vi "Settings Dialog.vi"(8 "error in (no error)":errorcluster caption="错误输入（无错误）", 11 "Settings in":T10={"Hardware Configuration"={"电压读取设置"={"DAQmx Channel"="", "Max Input"=0.0, "Min Input"=0.0, "Sample Rate"=0.0, "Sample Number"=0, "DAQmx Task"="", "device in"=""}, "角度传感器设置"={"counter"="Dev1/ctr0", "units"=10146, "分辨率"=0, "初始角度"=0.0, "DecodingType"=10092, "A相端口"="/Dev1/PFI8", "B相端口"="/Dev1/PFI8", "task in"=""}}, "Logging Configuration"={"Log File Base Path"=path "", "电压传感器转换率"=[], "电压传感器本底"=[]}, "Action Configuration"={"PLC设置"={"ActLogicalStationNumber"=9600, "ActUtlType"=refnum}, "动作设置"={"自动跳法测试动作"={"夹紧/松阀总"={"变量类型"=2, "PLC地址"=0, "size"=0, "写入数据(写入时有效)"=0}, "夹紧/松阀齿"={"变量类型"=2, "PLC地址"=0, "size"=0, "写入数据(写入时有效)"=0}, "方向机供油"={"变量类型"=2, "PLC地址"=0, "size"=0, "写入数据(写入时有效)"=0}, "扭杆紧/松"={"变量类型"=2, "PLC地址"=0, "size"=0, "写入数据(写入时有效)"=0}, "电机使能"={"变量类型"=2, "PLC地址"=0, "size"=0, "写入数据(写入时有效)"=0}, "内泄漏开"={"变量类型"=2, "PLC地址"=0, "size"=0, "写入数据(写入时有效)"=0}, "内泄漏停"={"变量类型"=2, "PLC地址"=0, "size"=0, "写入数据(写入时有效)"=0}, "数控钻孔启动"={"变量类型"=2, "PLC地址"=0, "size"=0, "写入数据(写入时有效)"=0}, "托起缸上"={"变量类型"=2, "PLC地址"=0, "size"=0, "写入数据(写入时有效)"=0}, "托起缸下"={"变量类型"=2, "PLC地址"=0, "size"=0, "写入数据(写入时有效)"=0}, "连续压紧开"={"变量类型"=2, "PLC地址"=0, "size"=0, "写入数据(写入时有效)"=0}, "连续压紧关"={"变量类型"=2, "PLC地址"=0, "size"=0, "写入数据(写入时有效)"=0}, "上上限启动"={"变量类型"=2, "PLC地址"=0, "size"=0, "写入数据(写入时有效)"=0}, "上限启动"={"变量类型"=2, "PLC地址"=0, "size"=0, "写入数据(写入时有效)"=0}, "压销自动"={"变量类型"=2, "PLC地址"=0, "size"=0, "写入数据(写入时有效)"=0}, "压销"={"变量类型"=2, "PLC地址"=0, "size"=0, "写入数据(写入时有效)"=0}}, "其他动作"={"其他指令1"={"变量类型"=2, "PLC地址"=0, "size"=0, "写入数据(写入时有效)"=0}, "其他指令2"={"变量类型"=2, "PLC地址"=0, "size"=0, "写入数据(写入时有效)"=0}, "其他指令3"={"变量类型"=2, "PLC地址"=0, "size"=0, "写入数据(写入时有效)"=0}, "其他指令4"={"变量类型"=2, "PLC地址"=0, "size"=0, "写入数据(写入时有效)"=0}, "其他指令5"={"变量类型"=2, "PLC地址"=0, "size"=0, "写入数据(写入时有效)"=0}}}, "电机设置"={"counter"="0", "方向端口"="", "当前方向"=FALSE, "频率"=0.0, "DAQmx Task"="0"}, "所有测试电机转动逻辑"={"啮合测试电机转动逻辑"={"反转判断条件1"={"传感器序号"=0, "条件"=enum."小于", "值"=0.0, "条件判断时间间隔"=0}, "停止判断条件1"={"角度传感器序号"=0, "正转/反转"=enum."正转", "反转次数"=0, "停止角度"=0.0, "停止角度误差范围"=0.0}}, "退回测试电机转动逻辑"={"反转判断条件1"={"传感器序号"=0, "条件"=enum."小于", "值"=0.0, "条件判断时间间隔"=0}, "停止判断条件1"={"角度传感器序号"=0, "正转/反转"=enum."正转", "反转次数"=0, "停止角度"=0.0, "停止角度误差范围"=0.0}}, "功能测试电机转动逻辑"={"反转判断条件1"={"传感器序号"=0, "条件"=enum."小于", "值"=0.0, "条件判断时间间隔"=0}, "停止判断条件1"={"角度传感器序号"=0, "正转/反转"=enum."正转", "反转次数"=0, "停止角度"=0.0, "停止角度误差范围"=0.0}}, "力特性测试电机转动逻辑"={"反转判断条件1"={"传感器序号"=0, "条件"=enum."小于", "值"=0.0, "条件判断时间间隔"=0}, "停止判断条件1"={"角度传感器序号"=0, "正转/反转"=enum."正转", "反转次数"=0, "停止角度"=0.0, "停止角度误差范围"=0.0}}, "自动调阀测试分中电机转动逻辑"={"反转判断条件1"={"传感器序号"=0, "条件"=enum."小于", "值"=0.0, "条件判断时间间隔"=0}, "停止判断条件1"={"角度传感器序号"=0, "正转/反转"=enum."正转", "反转次数"=0, "停止角度"=0.0, "停止角度误差范围"=0.0}}, "自动调阀测试对中电机转动逻辑"={"反转判断条件1"={"传感器序号"=0, "条件"=enum."小于", "值"=0.0, "条件判断时间间隔"=0}, "停止判断条件1"={"角度传感器序号"=0, "正转/反转"=enum."正转", "反转次数"=0, "停止角度"=0.0, "停止角度误差范围"=0.0}}, "内泄漏电机转动逻辑"={"反转判断条件1"={"传感器序号"=0, "条件"=enum."小于", "值"=0.0, "条件判断时间间隔"=0}, "停止判断条件1"={"角度传感器序号"=0, "正转/反转"=enum."正转", "反转次数"=0, "停止角度"=0.0, "停止角度误差范围"=0.0}}}}} caption="设置" {"Action Configuration"."动作设置"."其他动作"."其他指令5"."变量类型" items=["X", "Y", "M", "D"]; "Action Configuration"."动作设置"."其他动作"."其他指令4"."变量类型" items=["X", "Y", "M", "D"]; "Action Configuration"."动作设置"."其他动作"."其他指令3"."变量类型" items=["X", "Y", "M", "D"]; "Action Configuration"."动作设置"."其他动作"."其他指令2"."变量类型" items=["X", "Y", "M", "D"]; "Action Configuration"."动作设置"."其他动作"."其他指令1"."变量类型" items=["X", "Y", "M", "D"]; "Action Configuration"."动作设置"."自动跳法测试动作"."压销"."变量类型" items=["X", "Y", "M", "D"]; "Action Configuration"."动作设置"."自动跳法测试动作"."压销自动"."变量类型" items=["X", "Y", "M", "D"]; "Action Configuration"."动作设置"."自动跳法测试动作"."上限启动"."变量类型" items=["X", "Y", "M", "D"]; "Action Configuration"."动作设置"."自动跳法测试动作"."上上限启动"."变量类型" items=["X", "Y", "M", "D"]; "Action Configuration"."动作设置"."自动跳法测试动作"."连续压紧关"."变量类型" items=["X", "Y", "M", "D"]; "Action Configuration"."动作设置"."自动跳法测试动作"."连续压紧开"."变量类型" items=["X", "Y", "M", "D"]; "Action Configuration"."动作设置"."自动跳法测试动作"."托起缸下"."变量类型" items=["X", "Y", "M", "D"]; "Action Configuration"."动作设置"."自动跳法测试动作"."托起缸上"."变量类型" items=["X", "Y", "M", "D"]; "Action Configuration"."动作设置"."自动跳法测试动作"."数控钻孔启动"."变量类型" items=["X", "Y", "M", "D"]; "Action Configuration"."动作设置"."自动跳法测试动作"."内泄漏停"."变量类型" items=["X", "Y", "M", "D"]; "Action Configuration"."动作设置"."自动跳法测试动作"."内泄漏开"."变量类型" items=["X", "Y", "M", "D"]; "Action Configuration"."动作设置"."自动跳法测试动作"."电机使能"."变量类型" items=["X", "Y", "M", "D"]; "Action Configuration"."动作设置"."自动跳法测试动作"."扭杆紧/松"."变量类型" items=["X", "Y", "M", "D"]; "Action Configuration"."动作设置"."自动跳法测试动作"."方向机供油"."变量类型" items=["X", "Y", "M", "D"]; "Action Configuration"."动作设置"."自动跳法测试动作"."夹紧/松阀齿"."变量类型" items=["X", "Y", "M", "D"]; "Action Configuration"."动作设置"."自动跳法测试动作"."夹紧/松阀总"."变量类型" items=["X", "Y", "M", "D"]; "Hardware Configuration"."角度传感器设置"."DecodingType" items=["X1"=10090, "X2"=10091, "X4"=10092, "Two Pulse Counting"=10313]; "Hardware Configuration"."角度传感器设置"."units" items=["Degrees"=10146, "Radians"=10273, "Ticks"=10304, "From Custom Scale"=10065]}) -> (0 "error out":errorcluster caption="错误输出", 1 "Cancelled?":bool=TRUE caption="取消？", 2 "UI Refresh Needed?":bool caption="需要刷新UI？", 3 "Settings out":T10={"Hardware Configuration"={"电压读取设置"={"DAQmx Channel"="", "Max Input"=0.0, "Min Input"=0.0, "Sample Rate"=0.0, "Sample Number"=0, "DAQmx Task"="", "device in"=""}, "角度传感器设置"={"counter"="Dev1/ctr0", "units"=10146, "分辨率"=0, "初始角度"=0.0, "DecodingType"=10092, "A相端口"="/Dev1/PFI8", "B相端口"="/Dev1/PFI8", "task in"=""}}, "Logging Configuration"={"Log File Base Path"=path "", "电压传感器转换率"=[], "电压传感器本底"=[]}, "Action Configuration"={"PLC设置"={"ActLogicalStationNumber"=9600, "ActUtlType"=refnum}, "动作设置"={"自动跳法测试动作"={"夹紧/松阀总"={"变量类型"=2, "PLC地址"=0, "size"=0, "写入数据(写入时有效)"=0}, "夹紧/松阀齿"={"变量类型"=2, "PLC地址"=0, "size"=0, "写入数据(写入时有效)"=0}, "方向机供油"={"变量类型"=2, "PLC地址"=0, "size"=0, "写入数据(写入时有效)"=0}, "扭杆紧/松"={"变量类型"=2, "PLC地址"=0, "size"=0, "写入数据(写入时有效)"=0}, "电机使能"={"变量类型"=2, "PLC地址"=0, "size"=0, "写入数据(写入时有效)"=0}, "内泄漏开"={"变量类型"=2, "PLC地址"=0, "size"=0, "写入数据(写入时有效)"=0}, "内泄漏停"={"变量类型"=2, "PLC地址"=0, "size"=0, "写入数据(写入时有效)"=0}, "数控钻孔启动"={"变量类型"=2, "PLC地址"=0, "size"=0, "写入数据(写入时有效)"=0}, "托起缸上"={"变量类型"=2, "PLC地址"=0, "size"=0, "写入数据(写入时有效)"=0}, "托起缸下"={"变量类型"=2, "PLC地址"=0, "size"=0, "写入数据(写入时有效)"=0}, "连续压紧开"={"变量类型"=2, "PLC地址"=0, "size"=0, "写入数据(写入时有效)"=0}, "连续压紧关"={"变量类型"=2, "PLC地址"=0, "size"=0, "写入数据(写入时有效)"=0}, "上上限启动"={"变量类型"=2, "PLC地址"=0, "size"=0, "写入数据(写入时有效)"=0}, "上限启动"={"变量类型"=2, "PLC地址"=0, "size"=0, "写入数据(写入时有效)"=0}, "压销自动"={"变量类型"=2, "PLC地址"=0, "size"=0, "写入数据(写入时有效)"=0}, "压销"={"变量类型"=2, "PLC地址"=0, "size"=0, "写入数据(写入时有效)"=0}}, "其他动作"={"其他指令1"={"变量类型"=2, "PLC地址"=0, "size"=0, "写入数据(写入时有效)"=0}, "其他指令2"={"变量类型"=2, "PLC地址"=0, "size"=0, "写入数据(写入时有效)"=0}, "其他指令3"={"变量类型"=2, "PLC地址"=0, "size"=0, "写入数据(写入时有效)"=0}, "其他指令4"={"变量类型"=2, "PLC地址"=0, "size"=0, "写入数据(写入时有效)"=0}, "其他指令5"={"变量类型"=2, "PLC地址"=0, "size"=0, "写入数据(写入时有效)"=0}}}, "电机设置"={"counter"="0", "方向端口"="", "当前方向"=FALSE, "频率"=0.0, "DAQmx Task"="0"}, "所有测试电机转动逻辑"={"啮合测试电机转动逻辑"={"反转判断条件1"={"传感器序号"=0, "条件"=enum."小于", "值"=0.0, "条件判断时间间隔"=0}, "停止判断条件1"={"角度传感器序号"=0, "正转/反转"=enum."正转", "反转次数"=0, "停止角度"=0.0, "停止角度误差范围"=0.0}}, "退回测试电机转动逻辑"={"反转判断条件1"={"传感器序号"=0, "条件"=enum."小于", "值"=0.0, "条件判断时间间隔"=0}, "停止判断条件1"={"角度传感器序号"=0, "正转/反转"=enum."正转", "反转次数"=0, "停止角度"=0.0, "停止角度误差范围"=0.0}}, "功能测试电机转动逻辑"={"反转判断条件1"={"传感器序号"=0, "条件"=enum."小于", "值"=0.0, "条件判断时间间隔"=0}, "停止判断条件1"={"角度传感器序号"=0, "正转/反转"=enum."正转", "反转次数"=0, "停止角度"=0.0, "停止角度误差范围"=0.0}}, "力特性测试电机转动逻辑"={"反转判断条件1"={"传感器序号"=0, "条件"=enum."小于", "值"=0.0, "条件判断时间间隔"=0}, "停止判断条件1"={"角度传感器序号"=0, "正转/反转"=enum."正转", "反转次数"=0, "停止角度"=0.0, "停止角度误差范围"=0.0}}, "自动调阀测试分中电机转动逻辑"={"反转判断条件1"={"传感器序号"=0, "条件"=enum."小于", "值"=0.0, "条件判断时间间隔"=0}, "停止判断条件1"={"角度传感器序号"=0, "正转/反转"=enum."正转", "反转次数"=0, "停止角度"=0.0, "停止角度误差范围"=0.0}}, "自动调阀测试对中电机转动逻辑"={"反转判断条件1"={"传感器序号"=0, "条件"=enum."小于", "值"=0.0, "条件判断时间间隔"=0}, "停止判断条件1"={"角度传感器序号"=0, "正转/反转"=enum."正转", "反转次数"=0, "停止角度"=0.0, "停止角度误差范围"=0.0}}, "内泄漏电机转动逻辑"={"反转判断条件1"={"传感器序号"=0, "条件"=enum."小于", "值"=0.0, "条件判断时间间隔"=0}, "停止判断条件1"={"角度传感器序号"=0, "正转/反转"=enum."正转", "反转次数"=0, "停止角度"=0.0, "停止角度误差范围"=0.0}}}}} caption="设置" {"Action Configuration"."动作设置"."其他动作"."其他指令5"."变量类型" items=["X", "Y", "M", "D"]; "Action Configuration"."动作设置"."其他动作"."其他指令4"."变量类型" items=["X", "Y", "M", "D"]; "Action Configuration"."动作设置"."其他动作"."其他指令3"."变量类型" items=["X", "Y", "M", "D"]; "Action Configuration"."动作设置"."其他动作"."其他指令2"."变量类型" items=["X", "Y", "M", "D"]; "Action Configuration"."动作设置"."其他动作"."其他指令1"."变量类型" items=["X", "Y", "M", "D"]; "Action Configuration"."动作设置"."自动跳法测试动作"."压销"."变量类型" items=["X", "Y", "M", "D"]; "Action Configuration"."动作设置"."自动跳法测试动作"."压销自动"."变量类型" items=["X", "Y", "M", "D"]; "Action Configuration"."动作设置"."自动跳法测试动作"."上限启动"."变量类型" items=["X", "Y", "M", "D"]; "Action Configuration"."动作设置"."自动跳法测试动作"."上上限启动"."变量类型" items=["X", "Y", "M", "D"]; "Action Configuration"."动作设置"."自动跳法测试动作"."连续压紧关"."变量类型" items=["X", "Y", "M", "D"]; "Action Configuration"."动作设置"."自动跳法测试动作"."连续压紧开"."变量类型" items=["X", "Y", "M", "D"]; "Action Configuration"."动作设置"."自动跳法测试动作"."托起缸下"."变量类型" items=["X", "Y", "M", "D"]; "Action Configuration"."动作设置"."自动跳法测试动作"."托起缸上"."变量类型" items=["X", "Y", "M", "D"]; "Action Configuration"."动作设置"."自动跳法测试动作"."数控钻孔启动"."变量类型" items=["X", "Y", "M", "D"]; "Action Configuration"."动作设置"."自动跳法测试动作"."内泄漏停"."变量类型" items=["X", "Y", "M", "D"]; "Action Configuration"."动作设置"."自动跳法测试动作"."内泄漏开"."变量类型" items=["X", "Y", "M", "D"]; "Action Configuration"."动作设置"."自动跳法测试动作"."电机使能"."变量类型" items=["X", "Y", "M", "D"]; "Action Configuration"."动作设置"."自动跳法测试动作"."扭杆紧/松"."变量类型" items=["X", "Y", "M", "D"]; "Action Configuration"."动作设置"."自动跳法测试动作"."方向机供油"."变量类型" items=["X", "Y", "M", "D"]; "Action Configuration"."动作设置"."自动跳法测试动作"."夹紧/松阀齿"."变量类型" items=["X", "Y", "M", "D"]; "Action Configuration"."动作设置"."自动跳法测试动作"."夹紧/松阀总"."变量类型" items=["X", "Y", "M", "D"]; "Hardware Configuration"."角度传感器设置"."DecodingType" items=["X1"=10090, "X2"=10091, "X4"=10092, "Two Pulse Counting"=10313]; "Hardware Configuration"."角度传感器设置"."units" items=["Degrees"=10146, "Radians"=10273, "Ticks"=10304, "From Custom Scale"=10065]})   [LabVIEW 2015, in "Settings.lvlib"]
doc: "用于选择用户设置的对话框。"
uses:
  Settings.lvlib
  Acquisition/Hardware Configuration.ctl
  Settings.ctl
  Logging/Logging Configuration.ctl
  Action/Hardware Configuration.ctl
  <vilib>/Utility/xml.llb/Write to XML File(string).vi
  Acquisition/Acquisition.lvlib
  Logging/Logging.lvlib
  Action/Action.lvlib
panel:
  in  "Tab Control":T1(tab)
  in  "Hardware Configuration":T2={"电压读取设置"={"DAQmx Channel"="", "Max Input"=0.0, "Min Input"=0.0, "Sample Rate"=0.0, "Sample Number"=0, "DAQmx Task"="", "device in"=""}, "角度传感器设置"={"counter"="Dev1/ctr0", "units"=10146, "分辨率"=0, "初始角度"=0.0, "DecodingType"=10092, "A相端口"="/Dev1/PFI8", "B相端口"="/Dev1/PFI8", "task in"=""}} caption="硬件配置" {"角度传感器设置"."DecodingType" items=["X1"=10090, "X2"=10091, "X4"=10092, "Two Pulse Counting"=10313]; "角度传感器设置"."units" items=["Degrees"=10146, "Radians"=10273, "Ticks"=10304, "From Custom Scale"=10065]}
  in  "Logging Configuration":T3 caption="记录配置"
  in  "电机设置":T4={"counter"="Dev1/ctr0", "方向端口"="", "当前方向"=FALSE, "频率"=0.0, "DAQmx Task"=""} caption="电机配置"
  in  "PLC设置":T5={"ActLogicalStationNumber"=9600, "ActUtlType"=refnum}
  in  "啮合电机转动逻辑1":T6
  in  "退回电机转动逻辑1":T6
  in  "功能电机转动逻辑1":T6
  in  "力特性电机转动逻辑1":T6
  in  "Tab Control 2":enum32{"夹紧设置", "分中设置"}(tab)
  in  "夹紧PLC指令":T9={"变量类型"=2, "PLC地址"=0, "size"=0, "写入数据(写入时有效)"=0} {"变量类型" items=["X", "Y", "M", "D"]}
  in  "Cancel Button":bool caption="取消按钮"
  in  "OK Button":bool caption="确定按钮"
  # "设置"
  # "对话框不可见部分（用于连线板）"
  # "1、扭矩\n\n2、油压\n\n3、左推力\n\n4、右推力\n\n5、流量\n\n6、位移量"
  # "1、扭矩\n\n2、油压\n\n3、左推力\n\n4、右推力\n\n5、流量\n\n6、位移量"
  # "1、扭矩\n\n2、油压\n\n3、左推力\n\n4、右推力\n\n5、流量\n\n6、位移量"
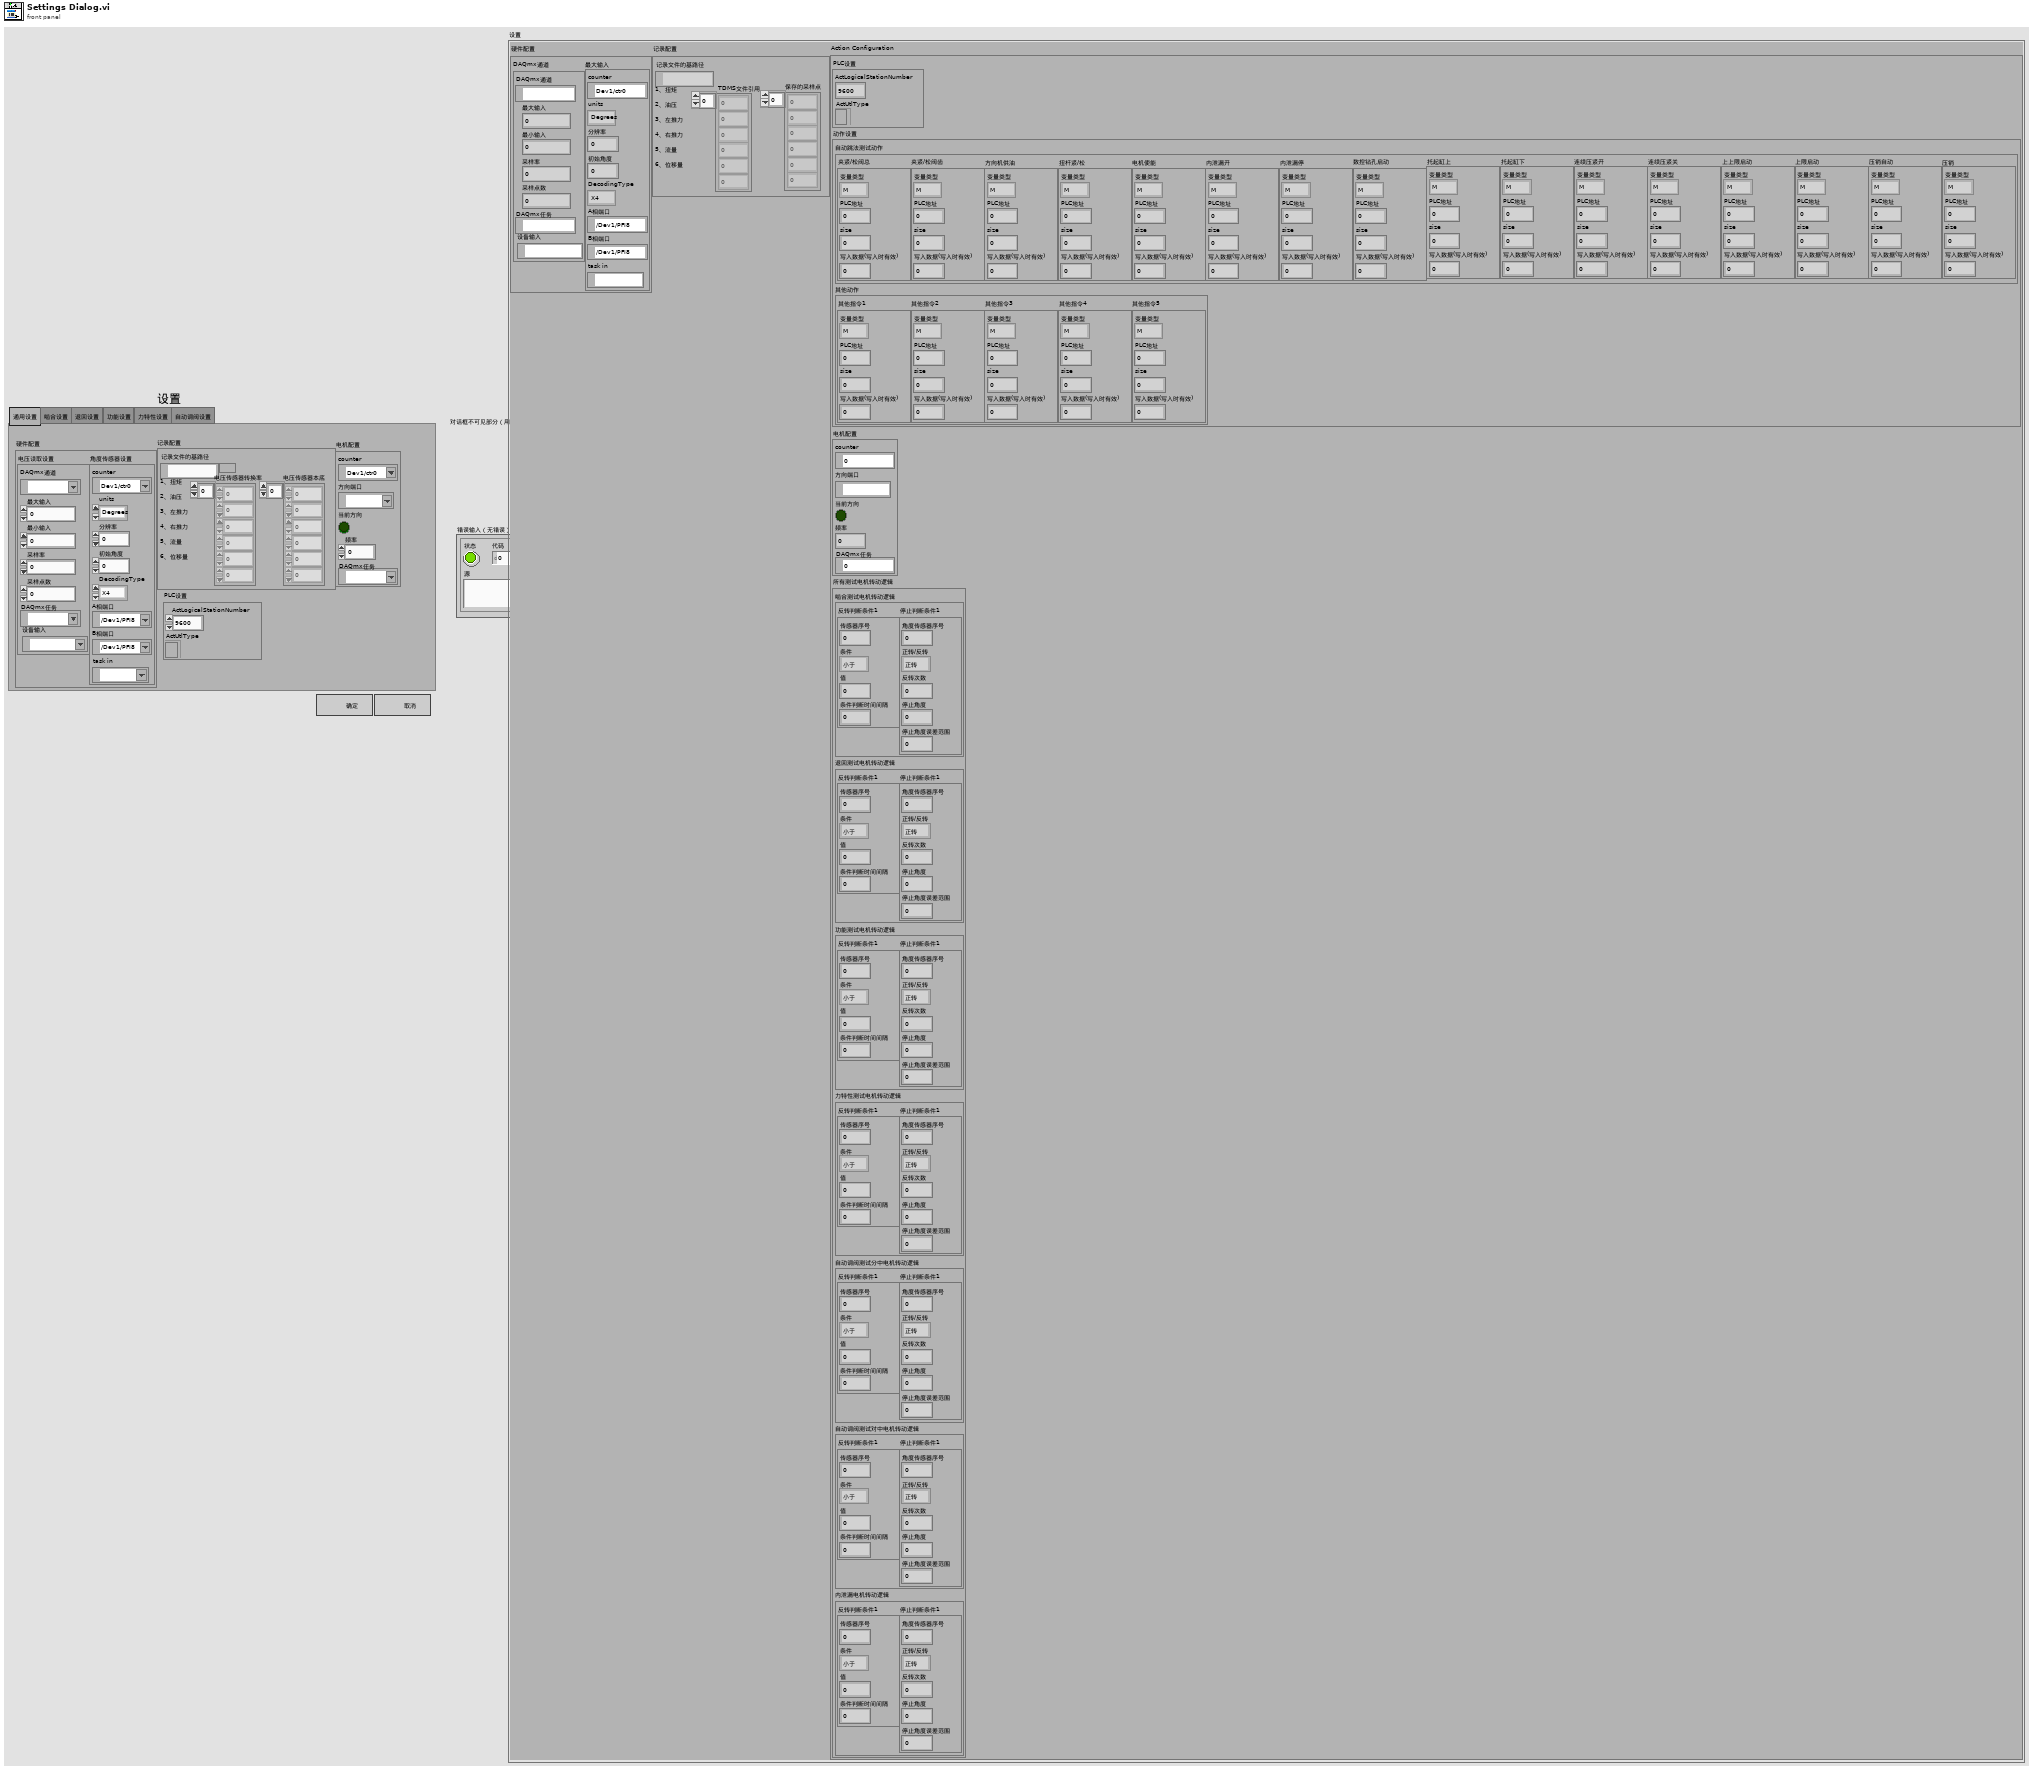
[diagram p1: front panel]
types:
  T1 = enum32{"通用设置", "啮合设置", "退回设置", "功能设置", "力特性设置", "自动调阀设置"}
  T2 = typedef "Acquisition.lvlib/Hardware Configuration.ctl" = cluster{"电压读取设置":cluster{"DAQmx Channel":tag, "Max Input":dbl, "Min Input":dbl, "Sample Rate":dbl, "Sample Number":i32, "DAQmx Task":refnum<k21>, "device in":tag}, "角度传感器设置":cluster{"counter":tag, "units":i32, "分辨率":i32, "初始角度":dbl, "DecodingType":i32, "A相端口":tag, "B相端口":tag, "task in":refnum<k21>}}
  T3 = typedef "Logging.lvlib/Logging Configuration.ctl" = cluster{"Log File Base Path":path, "电压传感器转换率":dbl[], "电压传感器本底":dbl[]}
  T4 = typedef "Action.lvlib/电机控制设置.ctl" = cluster{"counter":tag, "方向端口":tag, "当前方向":bool, "频率":dbl, "DAQmx Task":refnum<k21>}
  T5 = typedef "Action.lvlib/PLC设置.ctl" = cluster{"ActLogicalStationNumber":i32, "ActUtlType":refnum<k7>}
  T6 = typedef "Action.lvlib/电机转动逻辑1.ctl" = cluster{"反转判断条件1":T7, "停止判断条件1":T8}
  T7 = typedef "Action.lvlib/反转判断条件1.ctl" = cluster{"传感器序号":i32, "条件":enum16{"小于", "大于", "等于"}, "值":dbl, "条件判断时间间隔":i32}
  T8 = typedef "Action.lvlib/停止判断条件1.ctl" = cluster{"角度传感器序号":i32, "正转/反转":enum16{"正转", "反转"}, "反转次数":i32, "停止角度":dbl, "停止角度误差范围":dbl}
  T9 = typedef "Action.lvlib/PLC控制指令.ctl" = cluster{"变量类型":u32, "PLC地址":i32, "size":i32, "写入数据(写入时有效)":i16}
  T10 = typedef "Settings.lvlib/Settings.ctl" = cluster{"Hardware Configuration":T2, "Logging Configuration":T3, "Action Configuration":T11}
  T11 = typedef "Action.lvlib/Hardware Configuration.ctl" = cluster{"PLC设置":T5, "动作设置":T12, "电机设置":T4, "所有测试电机转动逻辑":T15}
  T12 = typedef "Action.lvlib/动作设置.ctl" = cluster{"自动跳法测试动作":T13, "其他动作":T14}
  T13 = typedef "Action.lvlib/自动调阀测试动作设置.ctl" = cluster{"夹紧/松阀总":T9, "夹紧/松阀齿":T9, "方向机供油":T9, "扭杆紧/松":T9, "电机使能":T9, "内泄漏开":T9, "内泄漏停":T9, "数控钻孔启动":T9, "托起缸上":T9, "托起缸下":T9, "连续压紧开":T9, "连续压紧关":T9, "上上限启动":T9, "上限启动":T9, "压销自动":T9, "压销":T9}
  T14 = typedef "Action.lvlib/其他动作设置 .ctl" = cluster{"其他指令1":T9, "其他指令2":T9, "其他指令3":T9, "其他指令4":T9, "其他指令5":T9}
  T15 = typedef "Action.lvlib/所有测试电机转动逻辑.ctl" = cluster{"啮合测试电机转动逻辑":T6, "退回测试电机转动逻辑":T6, "功能测试电机转动逻辑":T6, "力特性测试电机转动逻辑":T6, "自动调阀测试分中电机转动逻辑":T6, "自动调阀测试对中电机转动逻辑":T6, "内泄漏电机转动逻辑":T6}
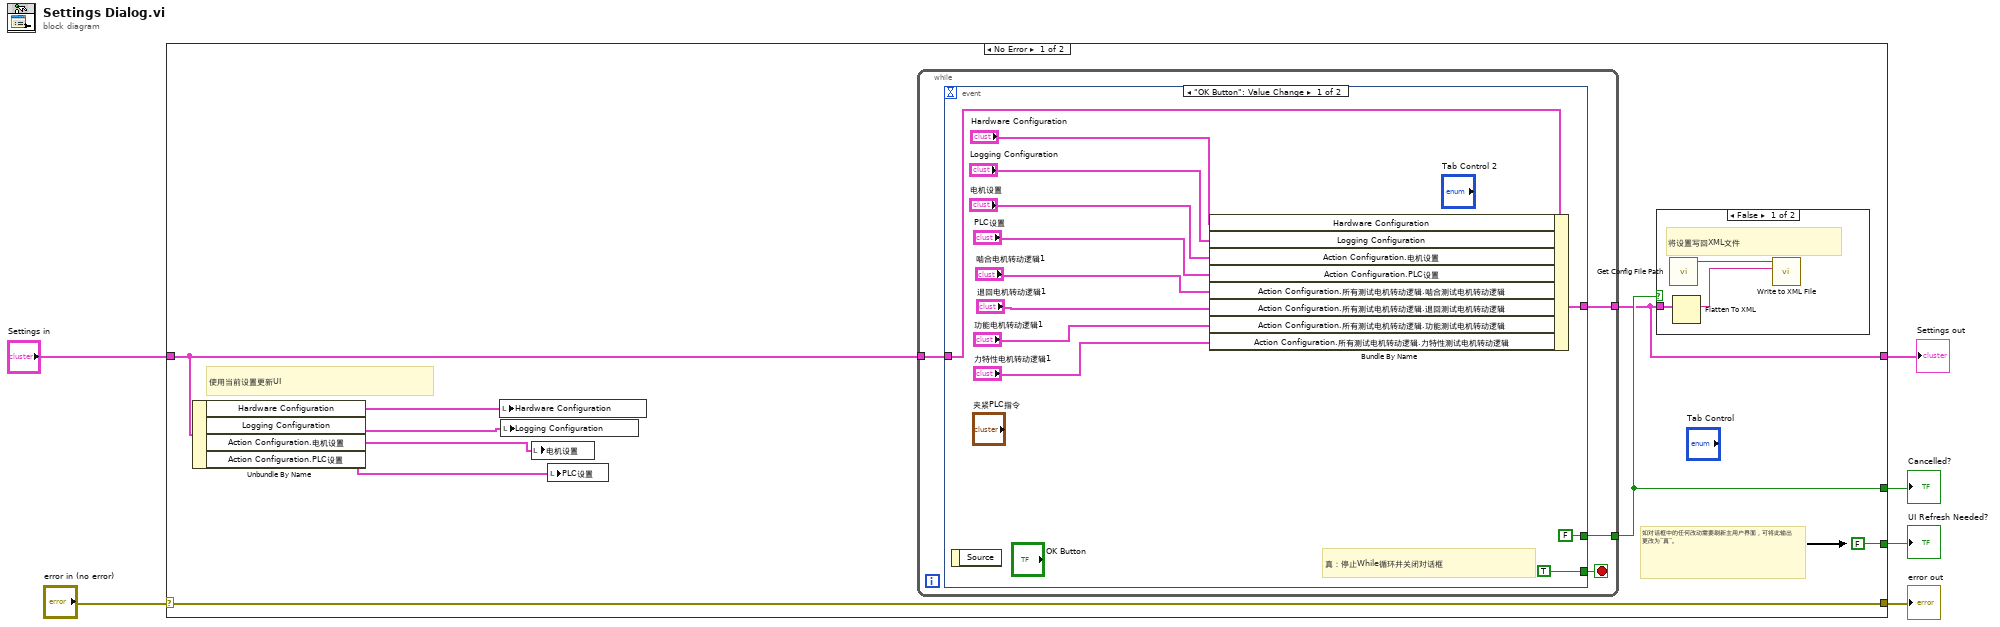
[diagram p0: block diagram]
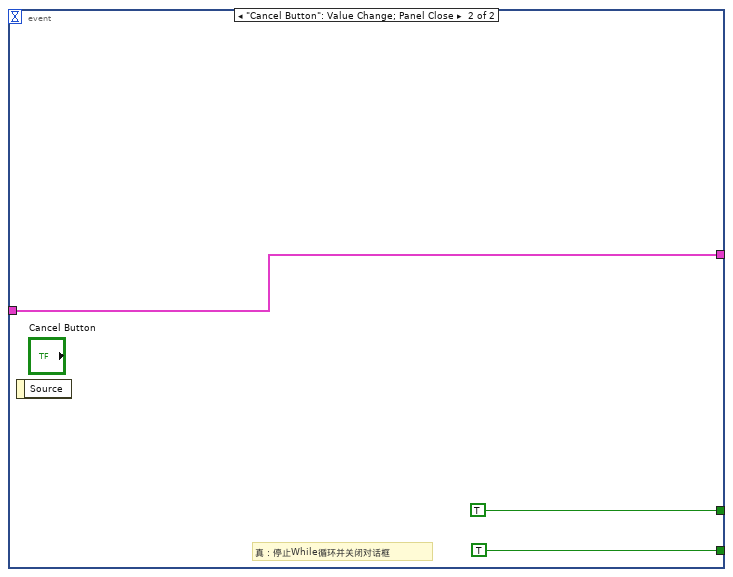
[diagram p2: hidden frame]
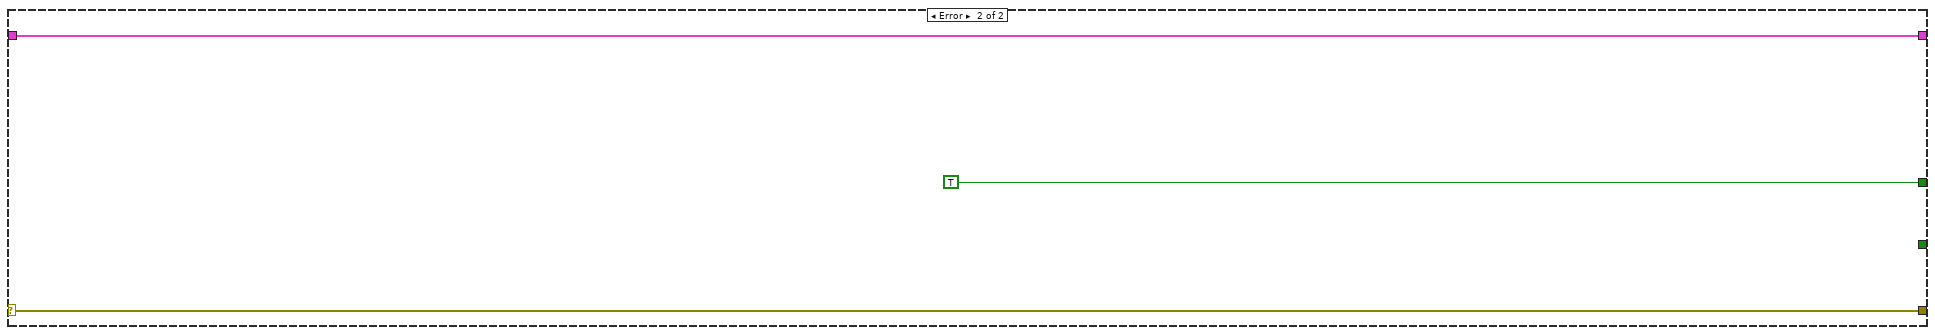
[diagram p4: hidden frame]
diagram:
  n1 = case shown="No Error" "error in (no error)" {
    selector: "error in (no error)" -> [w15 w40]
    tunnel: [w15 w40] -> w6
    tunnel: "Settings in" -> [w11 w39]
    tunnel: [w12 w39] -> w1
    tunnel: [FALSE ("UI Refresh Needed?") _] -> w5
    tunnel: [w13 TRUE ("UI Refresh Needed?")] -> w4
    frame No Error {
      # "使用当前设置更新UI"
      # "如对话框中的任何改动需要刷新主用户界面，可将此输出更改为“真”。"
      n2 = Unbundle By Name(w11) -> ("Hardware Configuration"=w10:T2, "Logging Configuration"=w9:T3, "Action Configuration.电机设置"=w8:T4, "Action Configuration.PLC设置"=w7:T5)
      n3 = local write "Hardware Configuration"(w10) -> ()
      n4 = local write "Logging Configuration"(w9) -> ()
      n5 = local write "电机设置"(w8) -> ()
      n6 = local write "PLC设置"(w7) -> ()
      n7 = while {
        tunnel: [w19] -> w13
        tunnel: [w18] -> w12
        tunnel: w11 -> [w17]
        stop <- w16 stop-if-true
        n8 = event shown="[0] \"OK Button\": Value Change" {
          selector: _ -> [_ _]
          dyn-events: _ -> [_ _]
          timeout: _ -> [_ _]
          tunnel: [w29 w34] -> w18
          tunnel: w17 -> [w28 w34]
          tunnel: [FALSE ("UI Refresh Needed?") TRUE ("UI Refresh Needed?")] -> w19
          tunnel: [TRUE TRUE] -> w16
          event "OK Button": Value Change {
            # "真：停止While循环并关闭对话框"
            n9 = event-data() -> ()  [unwired: 1 in, 1 out]
            n10 = Bundle By Name(cluster=w28, "Hardware Configuration"="Hardware Configuration", "Logging Configuration"="Logging Configuration", "Action Configuration.电机设置"="电机设置", "Action Configuration.PLC设置"="PLC设置", "Action Configuration.所有测试电机转动逻辑.啮合测试电机转动逻辑"="啮合电机转动逻辑1", "Action Configuration.所有测试电机转动逻辑.退回测试电机转动逻辑"="退回电机转动逻辑1", "Action Configuration.所有测试电机转动逻辑.功能测试电机转动逻辑"="功能电机转动逻辑1", "Action Configuration.所有测试电机转动逻辑.力特性测试电机转动逻辑"="力特性电机转动逻辑1") -> (w29:T10)
          }
          event "Cancel Button": Value Change; Panel Close {
            # "真：停止While循环并关闭对话框"
            n11 = event-data() -> ()  [unwired: 1 in, 1 out]
          }
        }
      }
      n12 = case shown="False" w13 {
        tunnel: w12 -> [w36 _]
        frame False {
          # "将设置写回XML文件"
          n13 = call "Get Config File Path.vi"() -> ("XML File Path"=w37:path)  [unwired: 10 in, 1 out]
          n14 = Flatten To XML(anything=w36) -> (xml string=w35:string)
          n15 = call-poly <vilib>:"Write to XML File.vi"("XML Input"=w35, "XML File Path"=w37) -> ()  [unwired: 7 in, 3 out]
        }
        frame True {
        }
      }
    }
    frame Error {
    }
  }
  "UI Refresh Needed?" <- w5
  "error out" <- w6
  "Cancelled?" <- w4
  "Settings out" <- w1
